vi "setLvLib.vi"(8 "error in (no error)":errorcluster, 10 "pathLvLib":path, 11 "LibReader in":refnum<class "LibReader.lvclass">) -> (0 "error out":errorcluster, 3 "LibReader out":refnum<class "LibReader.lvclass">)   [LabVIEW 2018, in "LibReader.lvclass"]
doc: "Set the LabVIEW library."
uses:
  LibReader.lvclass
  LibReader.lvclass/LibReader.ctl
  <vilib>/regexp/Match Regular Expression.xnode
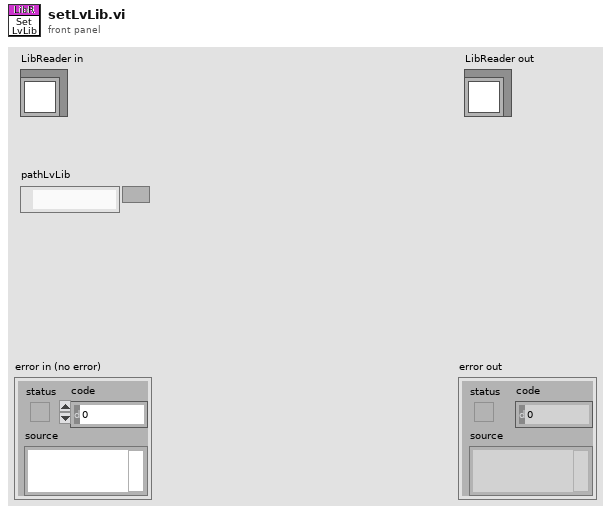
[diagram p1: front panel]
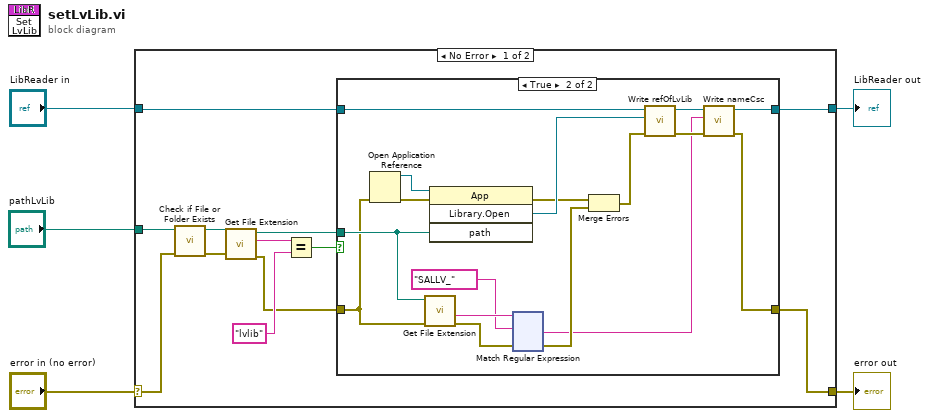
[diagram p0: block diagram]
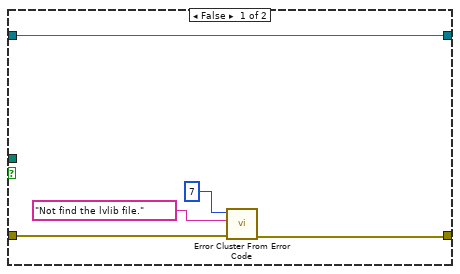
[diagram p2: hidden frame]
diagram:
  n1 = case shown="No Error" "error in (no error)" {
    selector: "error in (no error)" -> [w15 w155]
    tunnel: [w17 w155] -> w4
    tunnel: [w7 w154] -> w2
    tunnel: "LibReader in" -> [w8 w154]
    tunnel: "pathLvLib" -> [w16 _]
    frame No Error {
      n2 = call <vilib>:"Check if File or Folder Exists.vi"("error in (no error)"=w15, "path"=w16) -> ("error out"=w14:errorcluster, "dup path"=w13:path)  [unwired: 7 in, 1 out]
      n3 = call <vilib>:"Get File Extension.vi"("error in (no error)"=w14, "file"=w13) -> ("error out"=w6:errorcluster, "lowercase file extension"=w12:string, "dup file"=w10:path)  [unwired: 5 in, 2 out]
      n4 = Equal?(x=w12, y="lvlib") -> (x = y?=w9:bool)
      n5 = case shown="True" w9 {
        tunnel: [w20 w24] -> w17
        tunnel: w10 -> [_ w35]
        tunnel: w8 -> [w22 w36]
        tunnel: [w22 w25] -> w7
        tunnel: w6 -> [w21 w32]
        frame False {
          n6 = call <vilib>:"Error Cluster From Error Code.vi"("error in (no error)"=w21, "error message (\"\")"="Not find the lvlib file.", "error code (0)"=7) -> ("error out"=w20:errorcluster)  [unwired: 6 in]
        }
        frame True {
          n7 = Open Application Reference(8:w32) -> (0:w38:errorcluster, 3:w39:refnum<vi>)  [unwired: 3 in]
          n8 = call <vilib>:"Get File Extension.vi"("error in (no error)"=w32, "file"=w35) -> ("error out"=w31:errorcluster, "filename without extension"=w34:string)  [unwired: 5 in, 3 out]
          n9 = invoke class="App" method="Library.Open"(reference=w39, error in=w38, "path"=w35) -> (error out=w30:errorcluster, "Open Library"=w37:refnum<vi>)  [unwired: 1 in, 2 out]
          n10 = xnode "Match Regular Expression"("input string"=w34, "regular expression"="SALLV_", "error in"=w31) -> ("after match"=w23:string, "error out"=w29:errorcluster)  [unwired: 3 in, 3 out]
          n11 = Merge Errors(w30, w29) -> (w28:errorcluster)
          n12 = call "Write refOfLvLib.vi"("error in (no error)"=w28, "refOfLvLib"=w37, "LibReader in"=w36) -> ("error out"=w26:errorcluster, "LibReader out"=w27:refnum<class "LibReader.lvclass">)  [unwired: 7 in]
          n13 = call "Write nameCsc.vi"("error in (no error)"=w26, "nameCsc"=w23, "LibReader in"=w27) -> ("error out"=w24:errorcluster, "LibReader out"=w25:refnum<class "LibReader.lvclass">)  [unwired: 7 in]
        }
      }
    }
    frame Error {
    }
  }
  "error out" <- w4
  "LibReader out" <- w2
